vi "test Data Types (Integer Decoding).vi"(8 "error in (no error)":errorcluster, 11 "TestCase in":refnum<class "BCD.lvclass">) -> (0 "error out":errorcluster, 3 "TestCase out":refnum<class "BCD.lvclass">)   [LabVIEW 2027, in "BCD.lvclass"]
uses:
  BCD.lvclass
  5f41c702-736d-46cb-8ad7-d7a8da9834e5.vi
  e3375faa-55d5-40c5-9afa-67f8b88dd4b0.vi
  42a7bca9-d213-488f-a610-887b6bb38f81.vi
  b0f5f67f-c7b2-4b6f-9bdd-ee8cbe894007.vi
  eb865c1c-101d-43a3-aa66-c96ee64c9e7e.vi
  01ccdbfc-823f-4864-ac6e-0f9fb0e75310.vi
  0cc24d6e-6748-4204-8650-73a6176edd35.vi
  86949afa-0666-43c9-809e-5de6da9b4d1d.vi
  2d6e40c0-5fb9-4b9b-9465-c2daf76e77d7.vi
  031639a8-7589-4ff4-9d89-5a20bd13c62a.vi
  4902bbe7-6234-48da-b11f-73dcd207c588.vi
  62589f1a-0958-4038-a9e6-cbb235603fe5.vi
  841edd93-599c-498b-a273-a746ac5e7b71.vi
  93a7c20f-d3f7-4b01-b158-41e76f217b53.vi
  3a66866b-dca4-40cf-a6b6-ec7fa99c847f.vi
  705b34ac-4933-4895-9e10-b38a883783a7.vi
  8e77009d-e80f-487d-8924-5583bc157731.vi
  a43c630a-c30a-4052-b5ec-77f13c5d82c2.vi
  5f41c702-736d-46cb-8ad7-d7a8da9834e5.vi/136dcdcb-2dd3-4a4d-a796-a8f7a3f8e1ac.vi
  5f41c702-736d-46cb-8ad7-d7a8da9834e5.vi/a54b505c-1216-4ef4-8378-3ceda9d188df.vi
  Source/Get Bits Per Digit from Base.vi
  42a7bca9-d213-488f-a610-887b6bb38f81.vi/136dcdcb-2dd3-4a4d-a796-a8f7a3f8e1ac.vi
  42a7bca9-d213-488f-a610-887b6bb38f81.vi/a54b505c-1216-4ef4-8378-3ceda9d188df.vi
  eb865c1c-101d-43a3-aa66-c96ee64c9e7e.vi/136dcdcb-2dd3-4a4d-a796-a8f7a3f8e1ac.vi
  eb865c1c-101d-43a3-aa66-c96ee64c9e7e.vi/a54b505c-1216-4ef4-8378-3ceda9d188df.vi
  0cc24d6e-6748-4204-8650-73a6176edd35.vi/136dcdcb-2dd3-4a4d-a796-a8f7a3f8e1ac.vi
  0cc24d6e-6748-4204-8650-73a6176edd35.vi/a54b505c-1216-4ef4-8378-3ceda9d188df.vi
  2d6e40c0-5fb9-4b9b-9465-c2daf76e77d7.vi/136dcdcb-2dd3-4a4d-a796-a8f7a3f8e1ac.vi
  2d6e40c0-5fb9-4b9b-9465-c2daf76e77d7.vi/a54b505c-1216-4ef4-8378-3ceda9d188df.vi
  4902bbe7-6234-48da-b11f-73dcd207c588.vi/136dcdcb-2dd3-4a4d-a796-a8f7a3f8e1ac.vi
  4902bbe7-6234-48da-b11f-73dcd207c588.vi/a54b505c-1216-4ef4-8378-3ceda9d188df.vi
  841edd93-599c-498b-a273-a746ac5e7b71.vi/136dcdcb-2dd3-4a4d-a796-a8f7a3f8e1ac.vi
  841edd93-599c-498b-a273-a746ac5e7b71.vi/a54b505c-1216-4ef4-8378-3ceda9d188df.vi
  3a66866b-dca4-40cf-a6b6-ec7fa99c847f.vi/136dcdcb-2dd3-4a4d-a796-a8f7a3f8e1ac.vi
  3a66866b-dca4-40cf-a6b6-ec7fa99c847f.vi/a54b505c-1216-4ef4-8378-3ceda9d188df.vi
  C:/Program Files/National Instruments/LabVIEW 2027/vi.lib/addons/_JKI Toolkits/VI Tester/TestCase.llb/TestCase.lvclass
  <vilib>/addons/_JKI Toolkits/VI Tester/TestCase.llb/TestCase.lvclass
panel:
  out "BCD encoded value":bool[](array[boolean])
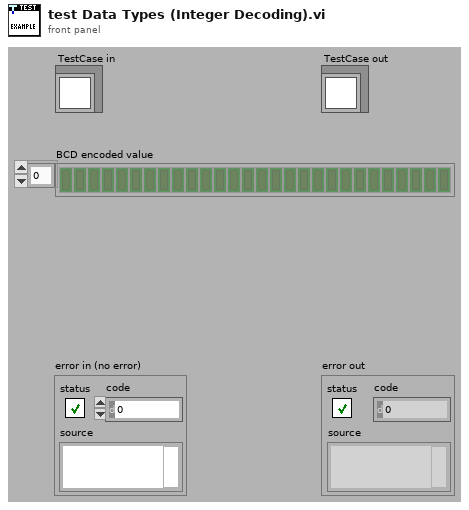
[diagram p1: front panel]
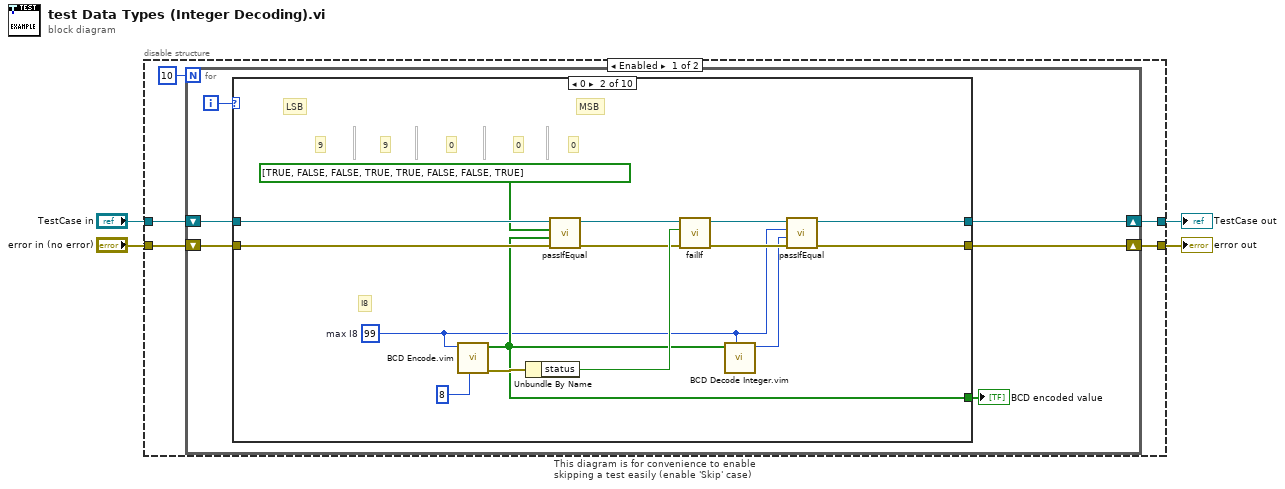
[diagram p0: block diagram]
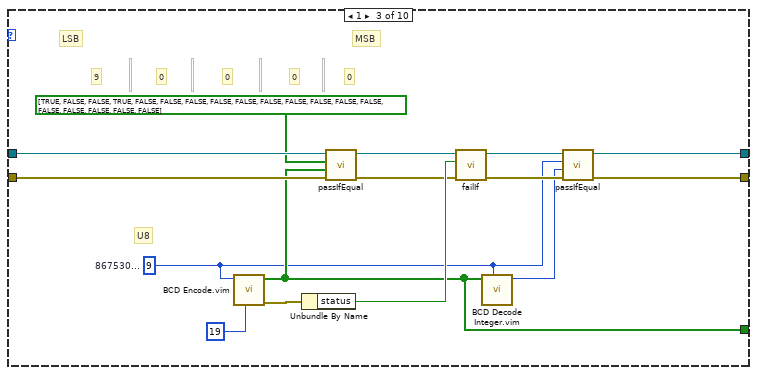
[diagram p3: hidden frame]
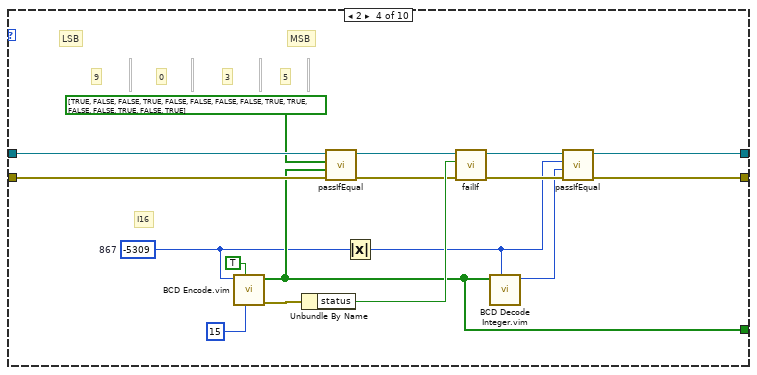
[diagram p4: hidden frame]
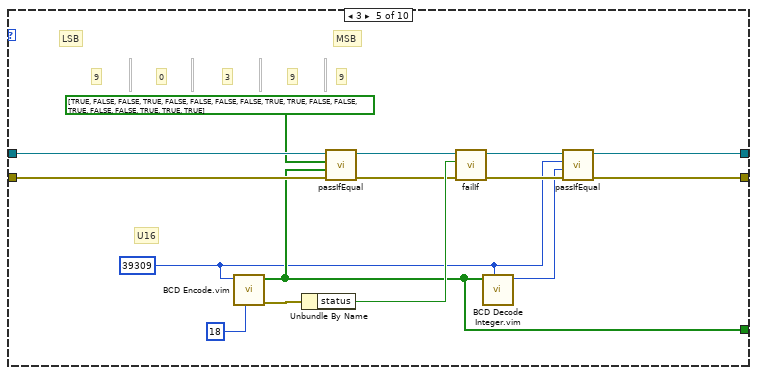
[diagram p5: hidden frame]
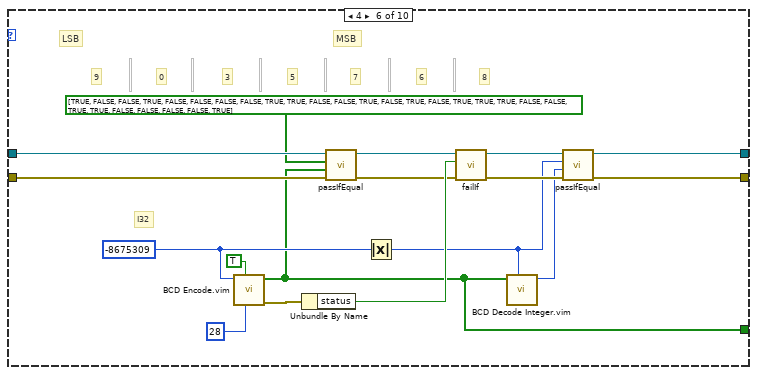
[diagram p6: hidden frame]
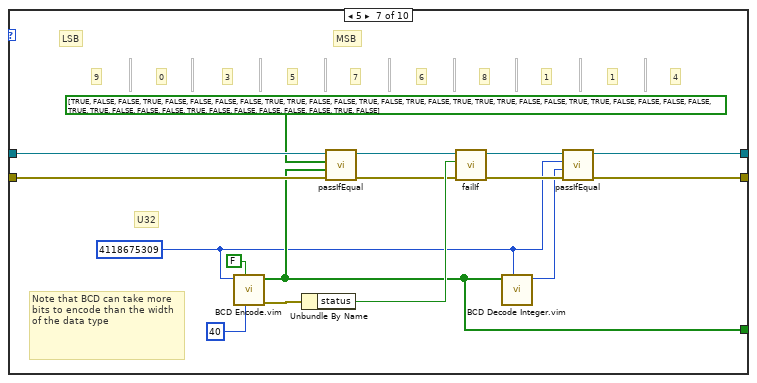
[diagram p7: hidden frame]
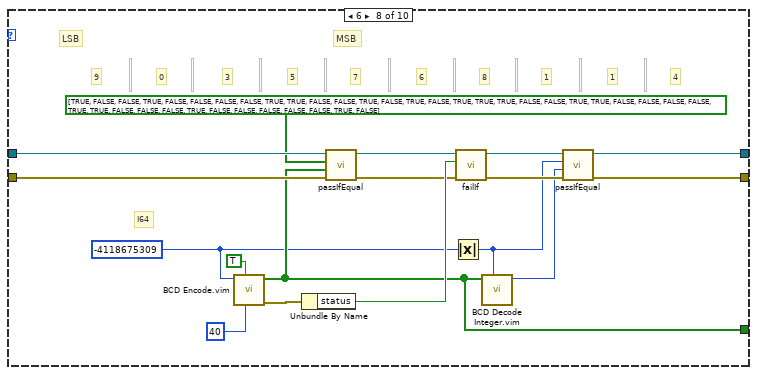
[diagram p8: hidden frame]
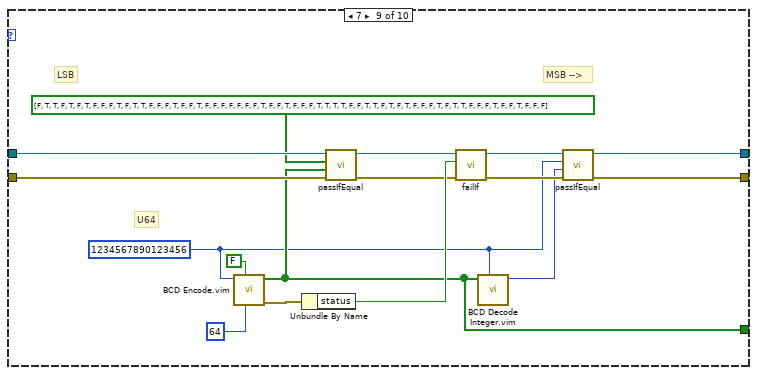
[diagram p9: hidden frame]
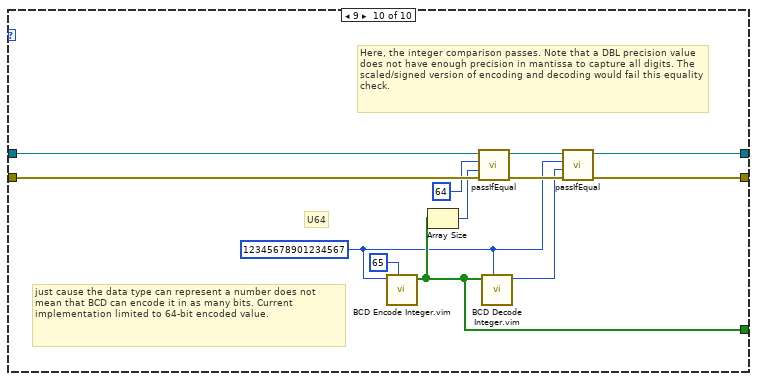
[diagram p10: hidden frame]
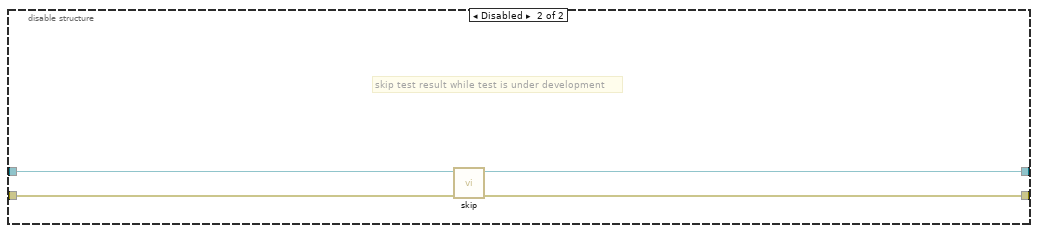
[diagram p11: hidden frame]
diagram:
  n1 = disable-structure "This diagram is for convenience to enable skipping a test easily (enable 'Skip' case)" shown="Enabled" {
    disable-tunnel: "TestCase in" -> [w9 w161]
    disable-tunnel: [w6 w159] -> w1
    disable-tunnel: [w7 w160] -> w3
    disable-tunnel: "error in (no error)" -> [w8 w158]
    frame Enabled {
      n2 = for {
        N: 10 -> [_]
        shift-right: [w12] -> w6
        shift-left: w9 -> [w15]
        shift-right: [w13] -> w7
        shift-left: w8 -> [w14]
        i -> [w11]
        n3 = case shown="0" w11 {
          tunnel: w15 -> [w17 w31 w46 w63 w78 w95 w111 w128 w144 w157]
          tunnel: w14 -> [w16 w30 w45 w62 w77 w94 w110 w127 w143 w156]
          tunnel: [w16 w22 w37 w54 w69 w85 w102 w119 w135 w153] -> w13
          tunnel: [w17 w21 w36 w53 w68 w84 w101 w118 w134 w152] -> w12
          tunnel: [_ w20 w35 w51 w67 w82 w99 w116 w133 w151] -> w10
          frame Default {
          }
          frame 0 {
            w18 = i8 99  # max I8
            # "I8"
            # "MSB"
            # "LSB"
            # "9"
            # "9"
            # "0"
            # "0"
            # "0"
            n4 = call "BCD Encode.vim"("data size (bits)"=8, "value"=w18) -> ("error out"=w28:errorcluster, "BCD encoded value"=w20:bool[])  [unwired: 7 in, 1 out]
            n5 = Unbundle By Name(w28) -> ("status"=w27:bool)
            n6 = call-dynamic "passIfEqual.vi"("error in (no error)"=w30, "y"=w20, "x"=bool[] [TRUE, FALSE, FALSE, TRUE, TRUE, FALSE, FALSE, TRUE] ("BCD encoded value"), "TestCase in"=w31) -> ("error out"=w25:errorcluster, "TestCase out"=w26:refnum<class "BCD.lvclass">)  [unwired: 6 in]
            n7 = call-dynamic "failIf.vi"("error in (no error)"=w25, "fail"=w27, "TestCase in"=w26) -> ("error out"=w23:errorcluster, "TestCase out"=w24:refnum<class "BCD.lvclass">)  [unwired: 7 in]
            n8 = call "BCD Decode Integer.vim"("expected value and type"=w18, "BCD encoded value"=w20) -> ("integer"=w19:i8)  [unwired: 9 in]
            n9 = call-dynamic "passIfEqual.vi"("error in (no error)"=w23, "y"=w19, "x"=w18, "TestCase in"=w24) -> ("error out"=w22:errorcluster, "TestCase out"=w21:refnum<class "BCD.lvclass">)  [unwired: 6 in]
          }
          frame 1 {
            w34 = u8 9  # 867530...
            # "U8"
            # "MSB"
            # "LSB"
            # "9"
            # "0"
            # "0"
            # "0"
            # "0"
            n10 = call "BCD Encode.vim"("data size (bits)"=19, "value"=w34) -> ("error out"=w43:errorcluster, "BCD encoded value"=w35:bool[])  [unwired: 7 in, 1 out]
            n11 = Unbundle By Name(w43) -> ("status"=w42:bool)
            n12 = call-dynamic "passIfEqual.vi"("error in (no error)"=w45, "y"=w35, "x"=bool[] [TRUE, FALSE, FALSE, TRUE, FALSE, FALSE, FALSE, FALSE, FALSE, FALSE, FALSE, FALSE, FALSE, FALSE, FALSE, FALSE, FALSE, FALSE, FALSE] ("BCD encoded value"), "TestCase in"=w46) -> ("error out"=w40:errorcluster, "TestCase out"=w41:refnum<class "BCD.lvclass">)  [unwired: 6 in]
            n13 = call-dynamic "failIf.vi"("error in (no error)"=w40, "fail"=w42, "TestCase in"=w41) -> ("error out"=w38:errorcluster, "TestCase out"=w39:refnum<class "BCD.lvclass">)  [unwired: 7 in]
            n14 = call "BCD Decode Integer.vim"("expected value and type"=w34, "BCD encoded value"=w35) -> ("integer"=w33:u8)  [unwired: 9 in]
            n15 = call-dynamic "passIfEqual.vi"("error in (no error)"=w38, "y"=w33, "x"=w34, "TestCase in"=w39) -> ("error out"=w37:errorcluster, "TestCase out"=w36:refnum<class "BCD.lvclass">)  [unwired: 6 in]
          }
          frame 2 {
            w50 = i16 -5309  # 867
            # "I16"
            # "MSB"
            # "LSB"
            # "9"
            # "0"
            # "3"
            # "5"
            n16 = call "BCD Encode.vim"("data size (bits)"=15, "signed"=TRUE, "value"=w50) -> ("error out"=w60:errorcluster, "BCD encoded value"=w51:bool[])  [unwired: 6 in, 1 out]
            n17 = Unbundle By Name(w60) -> ("status"=w59:bool)
            n18 = call-dynamic "passIfEqual.vi"("error in (no error)"=w62, "y"=w51, "x"=bool[] [TRUE, FALSE, FALSE, TRUE, FALSE, FALSE, FALSE, FALSE, TRUE, TRUE, FALSE, FALSE, TRUE, FALSE, TRUE] ("BCD encoded value"), "TestCase in"=w63) -> ("error out"=w57:errorcluster, "TestCase out"=w58:refnum<class "BCD.lvclass">)  [unwired: 6 in]
            n19 = Absolute Value(x=w50) -> (abs(x)=w48:i16)
            n20 = call-dynamic "failIf.vi"("error in (no error)"=w57, "fail"=w59, "TestCase in"=w58) -> ("error out"=w55:errorcluster, "TestCase out"=w56:refnum<class "BCD.lvclass">)  [unwired: 7 in]
            n21 = call "BCD Decode Integer.vim"("expected value and type"=w48, "BCD encoded value"=w51) -> ("integer"=w49:i16)  [unwired: 9 in]
            n22 = call-dynamic "passIfEqual.vi"("error in (no error)"=w55, "y"=w49, "x"=w48, "TestCase in"=w56) -> ("error out"=w54:errorcluster, "TestCase out"=w53:refnum<class "BCD.lvclass">)  [unwired: 6 in]
          }
          frame 3 {
            w65 = u16 39309 ("867...")
            # "9"
            # "U16"
            # "MSB"
            # "LSB"
            # "9"
            # "0"
            # "3"
            # "9"
            n23 = call "BCD Encode.vim"("data size (bits)"=18, "value"=w65) -> ("error out"=w75:errorcluster, "BCD encoded value"=w67:bool[])  [unwired: 7 in, 1 out]
            n24 = Unbundle By Name(w75) -> ("status"=w74:bool)
            n25 = call-dynamic "passIfEqual.vi"("error in (no error)"=w77, "y"=w67, "x"=bool[] [TRUE, FALSE, FALSE, TRUE, FALSE, FALSE, FALSE, FALSE, TRUE, TRUE, FALSE, FALSE, TRUE, FALSE, FALSE, TRUE, TRUE, TRUE] ("BCD encoded value"), "TestCase in"=w78) -> ("error out"=w72:errorcluster, "TestCase out"=w73:refnum<class "BCD.lvclass">)  [unwired: 6 in]
            n26 = call-dynamic "failIf.vi"("error in (no error)"=w72, "fail"=w74, "TestCase in"=w73) -> ("error out"=w70:errorcluster, "TestCase out"=w71:refnum<class "BCD.lvclass">)  [unwired: 7 in]
            n27 = call "BCD Decode Integer.vim"("expected value and type"=w65, "BCD encoded value"=w67) -> ("integer"=w66:u16)  [unwired: 9 in]
            n28 = call-dynamic "passIfEqual.vi"("error in (no error)"=w70, "y"=w66, "x"=w65, "TestCase in"=w71) -> ("error out"=w69:errorcluster, "TestCase out"=w68:refnum<class "BCD.lvclass">)  [unwired: 6 in]
          }
          frame 4 {
            w90 = -8675309 ("867...")
            # "8"
            # "6"
            # "7"
            # "I32"
            # "MSB"
            # "LSB"
            # "9"
            # "0"
            # "3"
            # "5"
            n29 = call "BCD Encode.vim"("data size (bits)"=28, "signed"=TRUE, "value"=w90) -> ("error out"=w92:errorcluster, "BCD encoded value"=w82:bool[])  [unwired: 6 in, 1 out]
            n30 = Unbundle By Name(w92) -> ("status"=w91:bool)
            n31 = call-dynamic "passIfEqual.vi"("error in (no error)"=w94, "y"=w82, "x"=bool[] [TRUE, FALSE, FALSE, TRUE, FALSE, FALSE, FALSE, FALSE, TRUE, TRUE, FALSE, FALSE, TRUE, FALSE, TRUE, FALSE, TRUE, TRUE, TRUE, FALSE, FALSE, TRUE, TRUE, FALSE, FALSE, FALSE, FALSE, TRUE] ("BCD encoded value"), "TestCase in"=w95) -> ("error out"=w88:errorcluster, "TestCase out"=w89:refnum<class "BCD.lvclass">)  [unwired: 6 in]
            n32 = Absolute Value(x=w90) -> (abs(x)=w81:i32)
            n33 = call-dynamic "failIf.vi"("error in (no error)"=w88, "fail"=w91, "TestCase in"=w89) -> ("error out"=w86:errorcluster, "TestCase out"=w87:refnum<class "BCD.lvclass">)  [unwired: 7 in]
            n34 = call "BCD Decode Integer.vim"("expected value and type"=w81, "BCD encoded value"=w82) -> ("integer"=w80:i32)  [unwired: 9 in]
            n35 = call-dynamic "passIfEqual.vi"("error in (no error)"=w86, "y"=w80, "x"=w81, "TestCase in"=w87) -> ("error out"=w85:errorcluster, "TestCase out"=w84:refnum<class "BCD.lvclass">)  [unwired: 6 in]
          }
          frame 5 {
            w97 = u32 4118675309 ("867...")
            # "Note that BCD can take more bits to encode than the width of the data type"
            # "4"
            # "1"
            # "1"
            # "8"
            # "6"
            # "7"
            # "U32"
            # "MSB"
            # "LSB"
            # "9"
            # "0"
            # "3"
            # "5"
            n36 = call "BCD Encode.vim"("data size (bits)"=40, "signed"=FALSE, "value"=w97) -> ("error out"=w108:errorcluster, "BCD encoded value"=w99:bool[])  [unwired: 6 in, 1 out]
            n37 = Unbundle By Name(w108) -> ("status"=w107:bool)
            n38 = call-dynamic "passIfEqual.vi"("error in (no error)"=w110, "y"=w99, "x"=bool[] [TRUE, FALSE, FALSE, TRUE, FALSE, FALSE, FALSE, FALSE, TRUE, TRUE, FALSE, FALSE, TRUE, FALSE, TRUE, FALSE, TRUE, TRUE, TRUE, FALSE, FALSE, TRUE, TRUE, FALSE, FALSE, FALSE, FALSE, TRUE, TRUE, FALSE, FALSE, FALSE, TRUE, FALSE, FALSE, FALSE, FALSE, FALSE, TRUE, FALSE] ("BCD encoded value"), "TestCase in"=w111) -> ("error out"=w105:errorcluster, "TestCase out"=w106:refnum<class "BCD.lvclass">)  [unwired: 6 in]
            n39 = call-dynamic "failIf.vi"("error in (no error)"=w105, "fail"=w107, "TestCase in"=w106) -> ("error out"=w103:errorcluster, "TestCase out"=w104:refnum<class "BCD.lvclass">)  [unwired: 7 in]
            n40 = call "BCD Decode Integer.vim"("expected value and type"=w97, "BCD encoded value"=w99) -> ("integer"=w98:u32)  [unwired: 9 in]
            n41 = call-dynamic "passIfEqual.vi"("error in (no error)"=w103, "y"=w98, "x"=w97, "TestCase in"=w104) -> ("error out"=w102:errorcluster, "TestCase out"=w101:refnum<class "BCD.lvclass">)  [unwired: 6 in]
          }
          frame 6 {
            w115 = i64 -4118675309 ("867...")
            # "4"
            # "1"
            # "1"
            # "8"
            # "6"
            # "7"
            # "I64"
            # "MSB"
            # "LSB"
            # "9"
            # "0"
            # "3"
            # "5"
            n42 = call "BCD Encode.vim"("data size (bits)"=40, "signed"=TRUE, "value"=w115) -> ("error out"=w125:errorcluster, "BCD encoded value"=w116:bool[])  [unwired: 6 in, 1 out]
            n43 = Unbundle By Name(w125) -> ("status"=w124:bool)
            n44 = call-dynamic "passIfEqual.vi"("error in (no error)"=w127, "y"=w116, "x"=bool[] [TRUE, FALSE, FALSE, TRUE, FALSE, FALSE, FALSE, FALSE, TRUE, TRUE, FALSE, FALSE, TRUE, FALSE, TRUE, FALSE, TRUE, TRUE, TRUE, FALSE, FALSE, TRUE, TRUE, FALSE, FALSE, FALSE, FALSE, TRUE, TRUE, FALSE, FALSE, FALSE, TRUE, FALSE, FALSE, FALSE, FALSE, FALSE, TRUE, FALSE] ("BCD encoded value"), "TestCase in"=w128) -> ("error out"=w122:errorcluster, "TestCase out"=w123:refnum<class "BCD.lvclass">)  [unwired: 6 in]
            n45 = Absolute Value(x=w115) -> (abs(x)=w113:i64)
            n46 = call-dynamic "failIf.vi"("error in (no error)"=w122, "fail"=w124, "TestCase in"=w123) -> ("error out"=w120:errorcluster, "TestCase out"=w121:refnum<class "BCD.lvclass">)  [unwired: 7 in]
            n47 = call "BCD Decode Integer.vim"("expected value and type"=w113, "BCD encoded value"=w116) -> ("integer"=w114:i64)  [unwired: 9 in]
            n48 = call-dynamic "passIfEqual.vi"("error in (no error)"=w120, "y"=w114, "x"=w113, "TestCase in"=w121) -> ("error out"=w119:errorcluster, "TestCase out"=w118:refnum<class "BCD.lvclass">)  [unwired: 6 in]
          }
          frame 7 {
            w131 = u64 1234567890123456 ("867...")
            # "U64"
            # "MSB -->"
            # "LSB"
            n49 = call "BCD Encode.vim"("data size (bits)"=64, "signed"=FALSE, "value"=w131) -> ("error out"=w141:errorcluster, "BCD encoded value"=w133:bool[])  [unwired: 6 in, 1 out]
            n50 = Unbundle By Name(w141) -> ("status"=w140:bool)
            n51 = call-dynamic "passIfEqual.vi"("error in (no error)"=w143, "y"=w133, "x"=bool[] [FALSE, TRUE, TRUE, FALSE, TRUE, FALSE, TRUE, FALSE, FALSE, FALSE, TRUE, FALSE, TRUE, TRUE, FALSE, FALSE, FALSE, TRUE, FALSE, FALSE, TRUE, FALSE, FALSE, FALSE, FALSE, FALSE, FALSE, FALSE, TRUE, FALSE, FALSE, TRUE, FALSE, FALSE, FALSE, TRUE, TRUE, TRUE, TRUE, FALSE, FALSE, TRUE, TRUE, FALSE, TRUE, FALSE, TRUE, FALSE, FALSE, FALSE, TRUE, FALSE, TRUE, TRUE, FALSE, FALSE, FALSE, TRUE, FALSE, FALSE, TRUE, FALSE, FALSE, FALSE] ("BCD encoded value"), "TestCase in"=w144) -> ("error out"=w138:errorcluster, "TestCase out"=w139:refnum<class "BCD.lvclass">)  [unwired: 6 in]
            n52 = call-dynamic "failIf.vi"("error in (no error)"=w138, "fail"=w140, "TestCase in"=w139) -> ("error out"=w136:errorcluster, "TestCase out"=w137:refnum<class "BCD.lvclass">)  [unwired: 7 in]
            n53 = call "BCD Decode Integer.vim"("expected value and type"=w131, "BCD encoded value"=w133) -> ("integer"=w130:u64)  [unwired: 9 in]
            n54 = call-dynamic "passIfEqual.vi"("error in (no error)"=w136, "y"=w130, "x"=w131, "TestCase in"=w137) -> ("error out"=w135:errorcluster, "TestCase out"=w134:refnum<class "BCD.lvclass">)  [unwired: 6 in]
          }
          frame 9 {
            w147 = u64 12345678901234567 ("867...")
            # "Here, the integer comparison passes. Note that a DBL precision value does not have enough precision in mantissa to capture all digits. The scaled/signed version of encoding and decoding would fail this equality check."
            # "just cause the data type can represent a number does not mean that BCD can encode it in as many bits. Current implementation limited to 64-bit encoded value."
            # "U64"
            n55 = call "BCD Encode Integer.vim"("data size (bits)"=65, "integer"=w147) -> ("BCD encoded value"=w151:bool[])  [unwired: 8 in, 1 out]
            n56 = Array Size(array=w151) -> (size(s)=w150:i32)
            n57 = call-dynamic "passIfEqual.vi"("error in (no error)"=w156, "y"=w150, "x"=64 ("size(s)"), "TestCase in"=w157) -> ("error out"=w154:errorcluster, "TestCase out"=w155:refnum<class "BCD.lvclass">)  [unwired: 6 in]
            n58 = call "BCD Decode Integer.vim"("expected value and type"=w147, "BCD encoded value"=w151) -> ("integer"=w146:u64)  [unwired: 9 in]
            n59 = call-dynamic "passIfEqual.vi"("error in (no error)"=w154, "y"=w146, "x"=w147, "TestCase in"=w155) -> ("error out"=w153:errorcluster, "TestCase out"=w152:refnum<class "BCD.lvclass">)  [unwired: 6 in]
          }
        }
        "BCD encoded value" <- w10
      }
    }
    frame Disabled {
      # "skip test result while test is under development"
      n60 = call <vilib>:"skip.vi"("error in (no error)"=w158, "TestCase in"=w161) -> ("error out"=w160:errorcluster, "TestCase out"=w159:refnum<class "BCD.lvclass">)  [unwired: 8 in]
    }
  }
  "error out" <- w3
  "TestCase out" <- w1
